vi "Part 1.vi"(10 "Iterations":i32=2, 11 "Input":string) -> (3 "Output":i64)   [LabVIEW 2021]
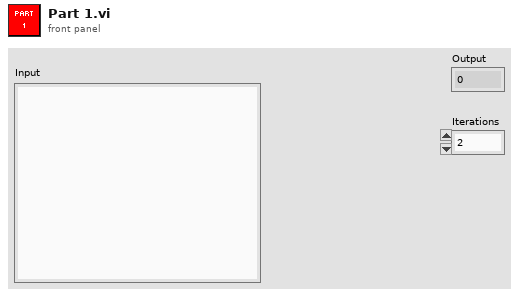
[diagram p1: front panel]
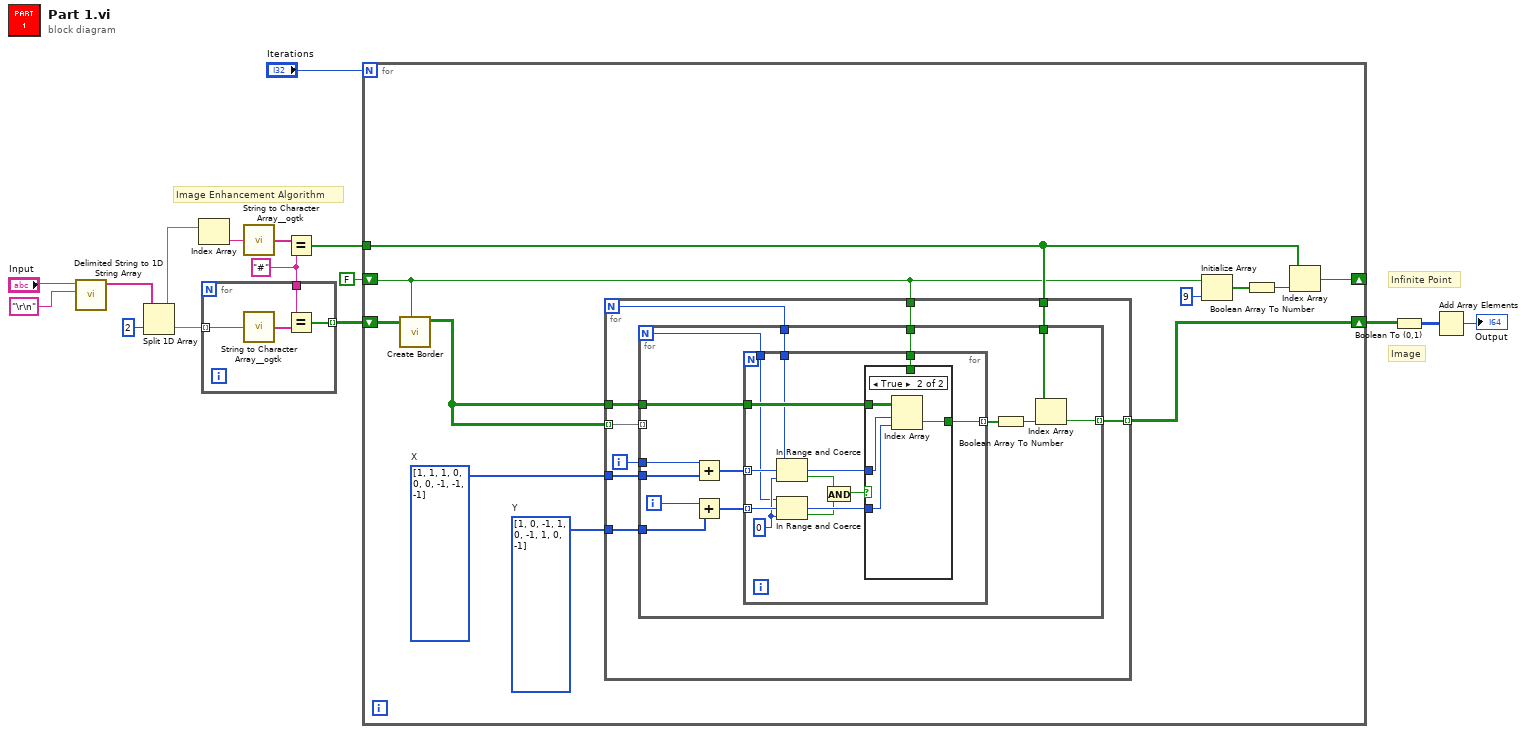
[diagram p0: block diagram]
diagram:
  w6 = "#"
  # "Image"
  # "Infinite Point"
  # "Image Enhancement Algorithm"
  n1 = call <vilib>:"Delimited String to 1D String Array.vi"("delimiter"="\r\n", "delimited string"="Input") -> ("string array"=w14:string[])  [unwired: 9 in]
  n2 = Split 1D Array(array=w14, index=2) -> (first subarray=w12:string[], second subarray=w7:string[])
  n3 = Index Array(array=w12) -> (element=w11:string)  [unwired: 1 in]
  n4 = for {
    tunnel: w7 -> [w19] mode=indexing
    tunnel: w6 -> [w18]
    tunnel: [w17] -> w5 mode=indexing
    n5 = call <userlib>:"String to Character Array__ogtk.vi"("Input String"=w19) -> ("Character Array"=w20:string[])
    n6 = Equal?(x=w18, y=w20) -> (x = y?=w17:bool[])
  }
  n7 = call <userlib>:"String to Character Array__ogtk.vi"("Input String"=w11) -> ("Character Array"=w10:string[])
  n8 = Equal?(x=w10, y=w6) -> (x = y?=w8:bool[])
  n9 = for {
    N: "Iterations" -> [_]
    shift-right: [w22] -> w3
    shift-left: w5 -> [w31]
    tunnel: w8 -> [w23]
    shift-right: [w27] -> _
    shift-left: FALSE -> [w21]
    w25 = i32[] [1, 1, 1, 0, 0, 0, -1, -1, -1]  # X
    w26 = i32[] [1, 0, -1, 1, 0, -1, 1, 0, -1]  # Y
    n10 = call "Create Border.vi"("Infinite Point"=w21, "Image In"=w31) -> ("Image Out"=w24:bool[][])  [unwired: 9 in]
    n11 = for {
      N -> [w32]
      tunnel: w24 -> [w40] mode=indexing
      tunnel: w25 -> [w38]
      tunnel: w26 -> [w37]
      tunnel: w24 -> [w36]
      tunnel: w23 -> [w35]
      tunnel: [w34] -> w22 mode=indexing
      tunnel: w21 -> [w33]
      i -> [w39]
      n12 = for {
        N -> [w42]
        tunnel: w40 -> [_] mode=indexing
        tunnel: w39 -> [w54]
        tunnel: w38 -> [w53]
        tunnel: w37 -> [w51]
        tunnel: w36 -> [w48]
        tunnel: w35 -> [w45]
        tunnel: [w44] -> w34 mode=indexing
        tunnel: w33 -> [w43]
        tunnel: w32 -> [w41]
        i -> [w52]
        n13 = Add(x=w54, y=w53) -> (x+y=w49:i32[])
        n14 = Add(x=w52, y=w51) -> (x+y=w50:i32[])
        n15 = for {
          tunnel: w50 -> [w61] mode=indexing
          tunnel: w49 -> [w62] mode=indexing
          tunnel: w48 -> [w63]
          tunnel: [w65] -> w47 mode=indexing
          tunnel: w43 -> [w64]
          tunnel: w42 -> [w56]
          tunnel: w41 -> [w55]
          w57 = 0 ("lower limit")
          n16 = In Range and Coerce(upper limit=w55, x=w62, lower limit=w57) -> (In Range?=w58:bool)  [unwired: 1 out]
          n17 = In Range and Coerce(upper limit=w56, x=w61, lower limit=w57) -> (In Range?=w59:bool)  [unwired: 1 out]
          n18 = And(x=w58, y=w59) -> (x .and. y?=w60:bool)
          n19 = case shown="True" w60 {
            tunnel: w63 -> [_ w70]
            tunnel: w62 -> [_ w69]
            tunnel: w61 -> [_ w68]
            tunnel: [w66 w67] -> w65
            tunnel: w64 -> [w66 _]
            frame False {
            }
            frame True {
              n20 = Index Array(array=w70, index (row)=w69, index (col)=w68) -> (element=w67:bool)
            }
          }
        }
        n21 = Boolean Array To Number(Boolean array=w47) -> (number=w46:u32)
        n22 = Index Array(array=w45, index=w46) -> (element=w44:bool)
      }
    }
    n23 = Initialize Array(w21, 9 ("dimension size")) -> (w29:bool[])
    n24 = Boolean Array To Number(Boolean array=w29) -> (number=w28:u32)
    n25 = Index Array(array=w23, index=w28) -> (element=w27:bool)
  }
  n26 = Boolean To (0,1)(Boolean=w3) -> (0, 1=w2:i16[][])
  n27 = Add Array Elements(numeric array=w2) -> (sum=→"Output":i16)
